vi "ServoMotor_slowMove.vi"(6 "Stop Button":bool, 7 "IO_Chanel":T1, 8 "Error In":errorcluster, 9 "pwm_target":dbl=0.0635, 11 "pwm_start":dbl=0.035) -> (0 "Error Out":errorcluster)   [LabVIEW 2019]
uses:
  WSCbot_V3_Toolkit.lvlibp/WSCBOTV3_Toolkit/IO/LowLevel/IO_Chanel_DIO.ctl
  <vilib>/Platform/TimedLoop/XDataNode/timing_clust.ctl
  <vilib>/Platform/TimedLoop/XDataNode/nitl_modes.ctl
  <vilib>/Platform/TimedLoop/XDataNode/wakeup.ctl
  WSCbot_V3_Toolkit.lvlibp/WSCBOTV3_Toolkit/IO/LowLevel/PWM.vi
  <vilib>/platform/TimedLoop/XDataNode/XDataNode.xnode
  WSCbot_V3_Toolkit.lvlibp
  <vilib>/Platform/TimedLoop/XDataNode/XDNodeRunTimeDep.lvlib
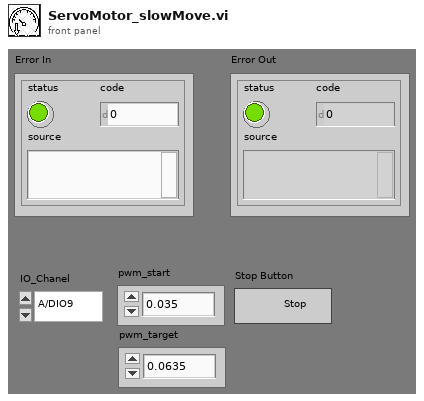
[diagram p1: front panel]
types:
  T1 = typedef "WSCbot_V3_Toolkit.lvlibp/IO_Chanel_DIO.ctl" = enum16{"A/DIO9", "A/DIO10", "C/DIO0", "C/DIO1", "C/DIO2", "C/DIO3", "C/DIO4", "C/DIO5", "C/DIO6"}
  T2 = typedef "XDNodeRunTimeDep.lvlib/timing_clust.ctl" = cluster{"Expected End [f-1]":u64, "Actual End [f-1]":u64, "Finished Late? [f-1]":bool, "Expected End [i-1]":u64, "Actual End [i-1]":u64, "Finished Late? [i-1]":bool, "Expected Start [i]":u64, "Actual Start [i]":u64, "Expected Start [f]":u64, "Actual Start [f]":u64, "Source Name":string, "Structure Name":string, "Period":i64, "Deadline":i64, "Offset":i64, "Start":i64, "Priority":i32, "Timeout":i32, "Mode":T3, "Wakeup Reason":T4, "Error":errorcluster, "Source Type":string, "Secondary Source Type":string, "Global End Time":u64, "Global Start Time":u64, "Frame Duration":u64, "Iteration Duration":u64, "Assigned CPU":i32, "I/O Scan Engine Mode":u32}
  T3 = typedef "XDNodeRunTimeDep.lvlib/nitl_modes.ctl" = enum32{"No Change", "Process missed periods, maintain original phase", "Discard missed periods, maintain original phase", "Process missed periods, ignore original phase", "Discard missed periods, ignore original phase"}
  T4 = typedef "XDNodeRunTimeDep.lvlib/wakeup.ctl" = enum32{"Normal", "Aborted", "Asynchronous wakeup", "Timing source error", "Timed loop error", "Timeout"}
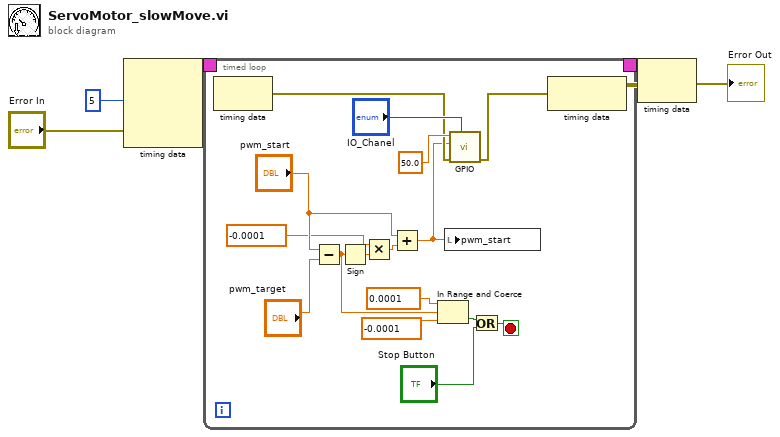
[diagram p0: block diagram]
diagram:
  n1 = node-c288(i64 5 ("Period"), "Error In") -> (w5:T2)  [unwired: 2 in]
  n2 = timed-loop {
    timing: w5 -> [_]
    timing-out: [_] -> w4
    stop <- w18 stop-if-true
    n3 = node-c288() -> (w16:errorcluster)  [unwired: 1 in]
    n4 = Subtract(x="pwm_start", y="pwm_target") -> (x-y=w8:dbl)
    n5 = Sign(1:w8) -> (0:w12:dbl)
    n6 = Multiply(x=-0.0001 ("y"), y=w12) -> (x*y=w11:dbl)
    n7 = Add(x="pwm_start", y=w11) -> (x+y=w10:dbl)
    n8 = In Range and Coerce(upper limit=0.0001, x=w8, lower limit=-0.0001) -> (In Range?=w19:bool)  [unwired: 1 out]
    n9 = local write "pwm_start"(w10) -> ()
    n10 = call-poly "GPIO.vi"("IO_Chanel"="IO_Chanel", "error in"=w16, "DutyCycle"=w10, "Frequency(Hz)"=50.0) -> ("error out"=w15:errorcluster)  [unwired: 7 in]
    n11 = Or(x=w19, y="Stop Button") -> (x .or. y?=w18:bool)
    n12 = node-c288(w15) -> ()  [unwired: 1 out]
  }
  n13 = node-c288(w4) -> (→"Error Out":errorcluster)
